vi "Get Connections for Inputs.vi"(8 "error in (no error)":errorcluster, 9 "Inputs":dbl[](array[numeric]), 10 "States Changed":bool[](array[boolean]), 11 "Routing Channel Configurations":T1[](array[typedef])) -> (0 "error out":errorcluster, 3 "Compiled Connections Indices":i32[](array[numeric]))   [LabVIEW 2020, in "Routing and Faulting Engine.lvlib"]
uses:
  Routing and Faulting Engine.lvlib
  Shared/Routing Channel Configuration.ctl
  Shared/Value-Connections Map.ctl
  Shared/Convert State Value to Integer.vi
  <vilib>/Utility/error.llb/Error Cluster From Error Code.vi
  Shared/Routing and Faulting Shared.lvlib
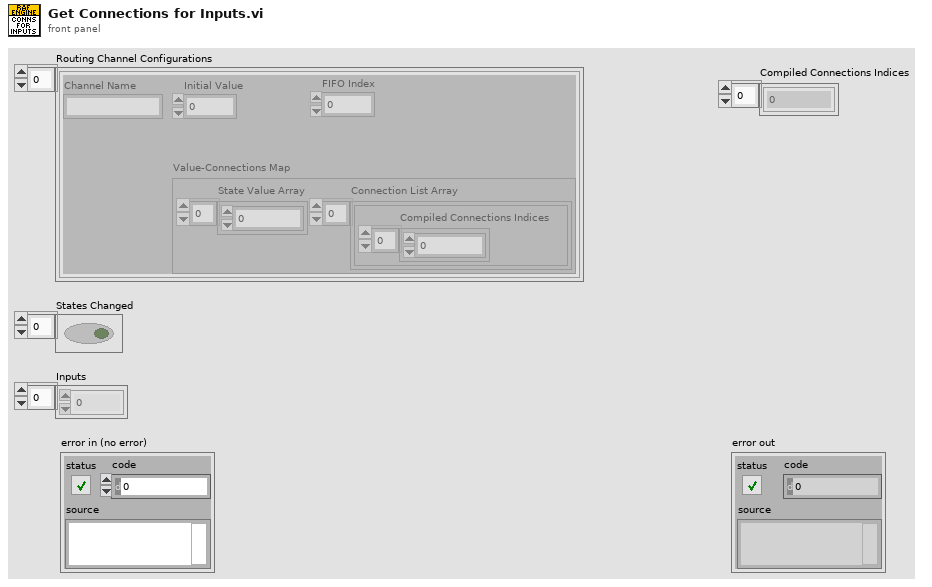
[diagram p1: front panel]
types:
  T1 = typedef "Routing and Faulting Shared.lvlib/Routing Channel Configuration.ctl" = cluster{"Channel Name":string, "Initial Value":dbl, "FIFO Index":i32, "Value-Connections Map":T2}
  T2 = typedef "Routing and Faulting Shared.lvlib/Value-Connections Map.ctl" = cluster{"State Value Array":i32[], "Connection List Array":cluster{"Compiled Connections Indices":i32[]}[]}
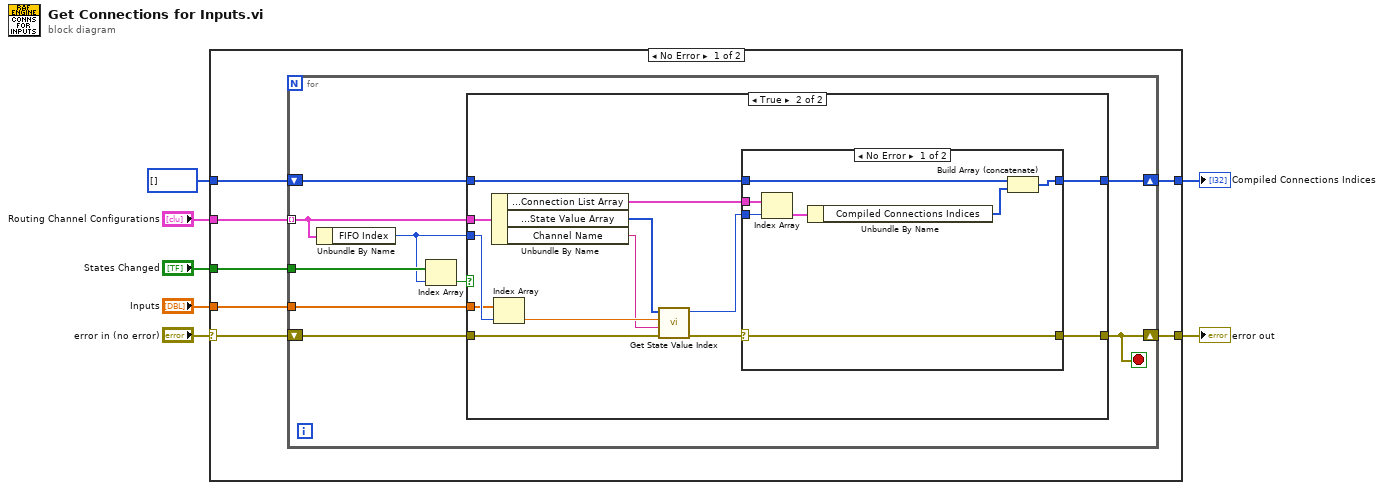
[diagram p0: block diagram]
diagram:
  n1 = case shown="No Error" "error in (no error)" {
    selector: "error in (no error)" -> [w11 w49]
    tunnel: "Inputs" -> [w14 _]
    tunnel: "States Changed" -> [w13 _]
    tunnel: "Routing Channel Configurations" -> [w12 _]
    tunnel: [w10 w49] -> w3
    tunnel: [w9 w48] -> w2
    tunnel: i32[] [] -> [w8 w48]
    frame No Error {
      n2 = for {
        tunnel: w13 -> [w22]
        tunnel: w12 -> [w23] mode=indexing
        tunnel: w14 -> [w20]
        shift-right: [w17] -> w10
        shift-left: w11 -> [w18]
        shift-right: [w15] -> w9
        shift-left: w8 -> [w16]
        stop <- w17 stop-if-true
        n3 = Unbundle By Name(w23) -> ("FIFO Index"=w19:i32)
        n4 = Index Array(array=w22, index=w19) -> (element=w21:bool)
        n5 = case shown="True" w21 {
          tunnel: w23 -> [_ w32]
          tunnel: w20 -> [_ w37]
          tunnel: w19 -> [_ w38]
          tunnel: w18 -> [w25 w31]
          tunnel: [w25 w36] -> w17
          tunnel: w16 -> [w24 w35]
          tunnel: [w24 w34] -> w15
          frame False {
            # "State didn't change. No connections."
          }
          frame True {
            n6 = Unbundle By Name(w32) -> ("Value-Connections Map.Connection List Array"=w33:cluster{"Compiled Connections Indices":i32[]}[], "Value-Connections Map.State Value Array"=w27:i32[], "Channel Name"=w26:string)
            n7 = Index Array(array=w37, index=w38) -> (element=w28:dbl)
            n8 = call "Get State Value Index.vi"("error in (no error)"=w31, "Channel Name"=w26, "State Value"=w28, "State Value Array"=w27) -> ("error out"=w30:errorcluster, "index of element"=w29:i32)  [unwired: 6 in]
            n9 = case shown="No Error" w30 {
              selector: w30 -> [w45 w46]
              tunnel: [w45 w46] -> w36
              tunnel: w29 -> [w43 _]
              tunnel: w33 -> [w42 _]
              tunnel: w35 -> [w41 w47]
              tunnel: [w40 w47] -> w34
              frame No Error {
                n10 = Index Array(array=w42, index=w43) -> (element=w44:cluster{"Compiled Connections Indices":i32[]})
                n11 = Unbundle By Name(w44) -> ("Compiled Connections Indices"=w39:i32[])
                n12 = Build Array (concatenate)(w41, w39) -> (w40:i32[])
              }
              frame Error {
              }
            }
          }
        }
      }
    }
    frame Error {
    }
  }
  "error out" <- w3
  "Compiled Connections Indices" <- w2
